vi "CU_openTrainFile.vi"(8 "error in (no error)":errorcluster, 10 "Path to XML file in":path caption="Path to XML document", 11 "ClassifierClass in":refnum<class "ClassifierClass.lvclass">) -> (0 "error out":errorcluster, 1 "CLass Labels out":string[](array[string]), 2 "Number of Trials out":i32, 3 "ClassifierClass out":refnum<class "ClassifierClass.lvclass">)   [LabVIEW 2016, in "Classifier.lvlib" / "ClassifierClass.lvclass"]
uses:
  ClassifierClass.lvclass
  ClassifierClass.lvclass/ClassifierClass.ctl
  <vilib>/xml/Load XML File.vi
  <vilib>/xml/NI_XML.lvlib
  _XML_EEG_Features/XML_EEG_Features.lvlib
panel:
  # "This VI is a part of BCI Design library, http://www.ru-bci.org \nCopyright © 2020, Sotnikov Peter, All rights reserved. License: CC BY-NC 4.0"
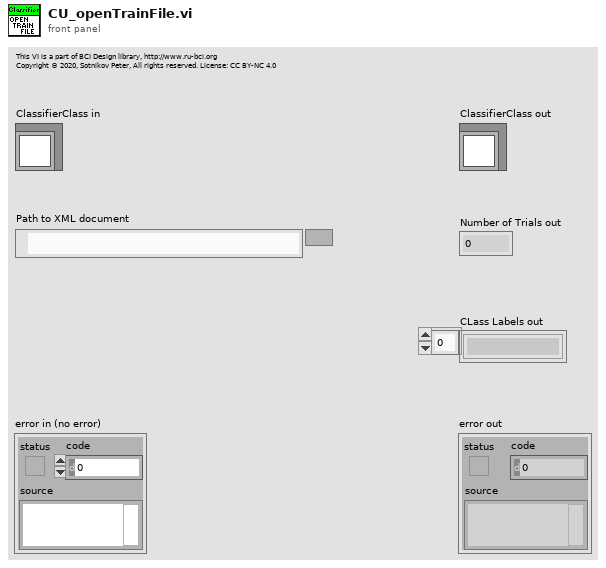
[diagram p1: front panel]
types:
  T1 = typedef "XML_EEG_Features.lvlib/XML_FF_Header.ctl" = cluster{"NumberOfTrials":i32, "NumberOfClasses":i32, "FeatureVectorLength":i32, "FeatureExtractionMethod":string}
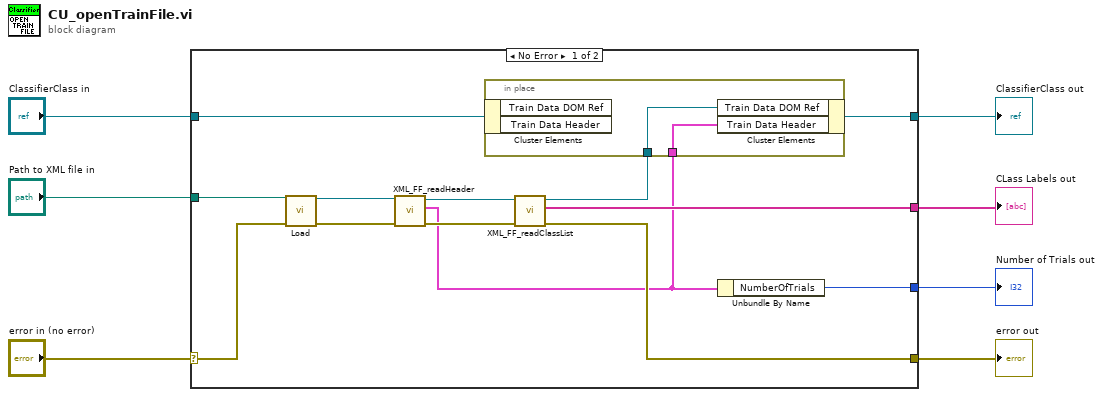
[diagram p0: block diagram]
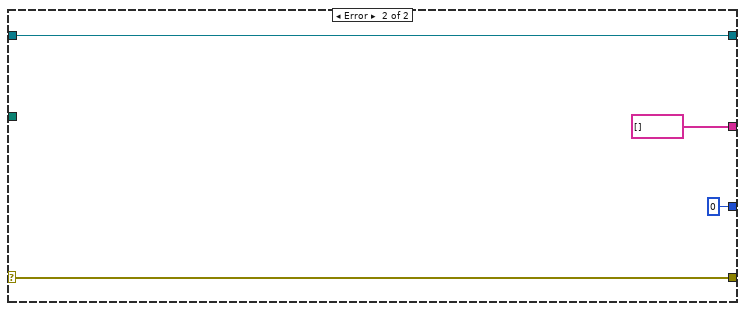
[diagram p2: hidden frame]
diagram:
  n1 = case shown="No Error" "error in (no error)" {
    selector: "error in (no error)" -> [w20 w26]
    tunnel: [w12 w26] -> w6
    tunnel: [w10 w25] -> w4
    tunnel: "ClassifierClass in" -> [w14 w25]
    tunnel: "Path to XML file in" -> [w17 _]
    tunnel: [w11 string[] [] ("CLassLabels out")] -> w2
    tunnel: [w9 0 ("NumberOfTrials")] -> w1
    frame No Error {
      n2 = call-poly <vilib>:"Load.vi"("path to XML document"=w17, "error in (no error)"=w20) -> ("DOM document out"=w19:refnum<k20>, "error out"=w18:errorcluster)  [unwired: 11 in, 1 out]
      n3 = call "XML_FF_readHeader.vi"("error in (no error)"=w18, "DOM document in"=w19) -> ("error out"=w16:errorcluster, "FF_Header out"=w8:T1, "DOM document out"=w15:refnum<k20>)  [unwired: 7 in]
      n4 = call "XML_FF_readClassList.vi"("error in (no error)"=w16, "DOM document in"=w15) -> ("error out"=w12:errorcluster, "CLassLabels out"=w11:string[], "DOM document out"=w13:refnum<k20>)  [unwired: 7 in]
      n5 = in-place {
        in-place-border: w13 -> [w22]
        in-place-border: w8 -> [w21]
        n6 = in-place-cluster #1(w14) -> ()  [unwired: 2 out]
        n7 = in-place-cluster #1("Train Data DOM Ref"=w22, "Train Data Header"=w21) -> (w10:refnum<class "ClassifierClass.lvclass">)
      }
      n8 = Unbundle By Name(w8) -> ("NumberOfTrials"=w9:i32)
    }
    frame Error {
    }
  }
  "error out" <- w6
  "ClassifierClass out" <- w4
  "CLass Labels out" <- w2
  "Number of Trials out" <- w1
